vi "solar_voy_def Export (Mods).vi"(10 "CMD":enum8{"CMD", "TLM"}(ring), 11 "MODIFIERS":T1) -> (3 "MODIFIERS_DEF":string)   [LabVIEW 2018]
doc: "This exports a COSMOS parameter/item modifier to string."
uses:
  solar_voy_def_ctl MODIFIERS UNITS.ctl
  solar_voy_def_ctl MODIFIERS STATE.ctl
  solar_voy_def_ctl MODIFIERS CONVERSION.ctl
  solar_voy_def_ctl MODIFIERS.ctl
  solar_voy_def_ctl MODIFIERS LIMITS.ctl
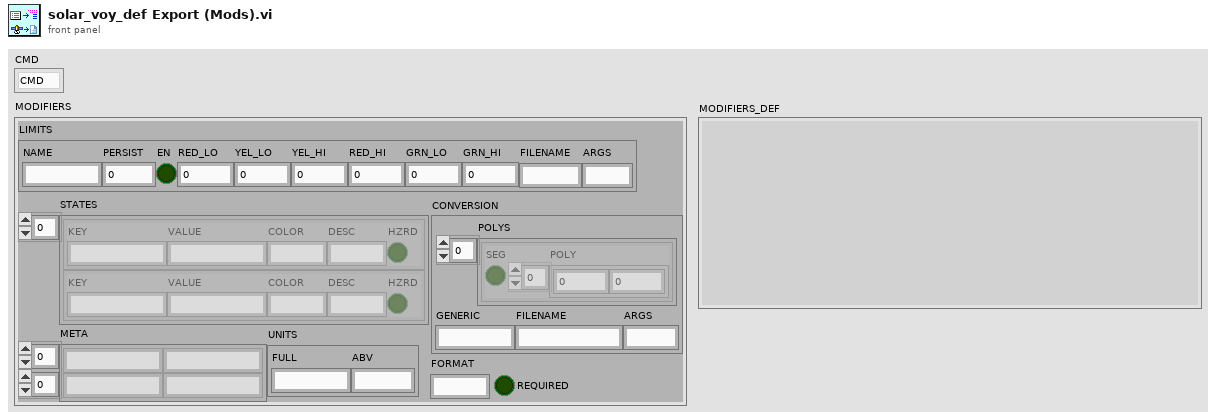
[diagram p1: front panel]
types:
  T1 = typedef "solar_voy_def_ctl MODIFIERS.ctl" = cluster{"LIMITS":T2, "UNITS":T3, "STATES":T4[], "CONVERSION":T5, "FORMAT":string, "REQUIRED":bool, "META":string[][]}
  T2 = typedef "solar_voy_def_ctl MODIFIERS LIMITS.ctl" = cluster{"NAME":string, "PERSIST":i32, "EN":bool, "RED_LO":dbl, "YEL_LO":dbl, "YEL_HI":dbl, "RED_HI":dbl, "GRN_LO":dbl, "GRN_HI":dbl, "FILENAME":string, "ARGS":string}
  T3 = typedef "solar_voy_def_ctl MODIFIERS UNITS.ctl" = cluster{"FULL":string, "ABV":string}
  T4 = typedef "solar_voy_def_ctl MODIFIERS STATE.ctl" = cluster{"KEY":string, "VALUE":string, "COLOR":string, "DESC":string, "HZRD":bool}
  T5 = typedef "solar_voy_def_ctl MODIFIERS CONVERSION.ctl" = cluster{"GENERIC":string, "FILENAME":string, "ARGS":string, "POLYS":cluster{"SEG":bool, "POLY":dbl[]}[]}
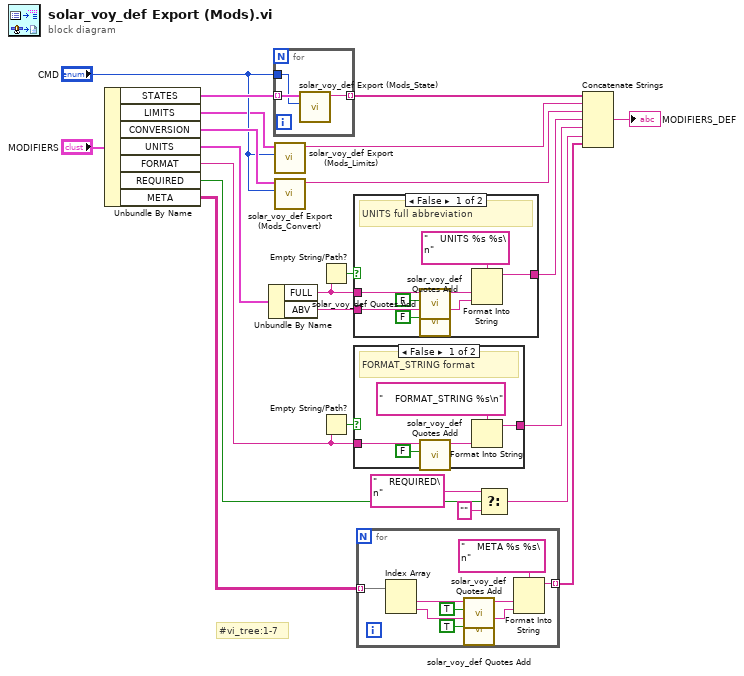
[diagram p0: block diagram]
diagram:
  # "#vi_tree:1-7"
  n1 = Unbundle By Name("MODIFIERS") -> ("STATES"=w22:T4[], "LIMITS"=w2:T2, "CONVERSION"=w19:T5, "UNITS"=w17:T3, "FORMAT"=w11:string, "REQUIRED"=w9:bool, "META"=w5:string[][])
  n2 = Unbundle By Name(w17) -> ("FULL"=w15:string, "ABV"=w14:string)
  n3 = for {
    tunnel: w22 -> [w25] mode=indexing
    tunnel: [w26] -> w21 mode=indexing
    tunnel: "CMD" -> [w24]
    n4 = call "solar_voy_def Export (Mods_State).vi"("CMD"=w24, "STATE"=w25) -> ("STATE_DEF"=w26:string)  [unwired: 9 in]
  }
  n5 = call "solar_voy_def Export (Mods_Limits).vi"("CMD"="CMD", "LIMITS"=w2) -> ("LIMITS_DEF"=w1:string)  [unwired: 9 in]
  n6 = call "solar_voy_def Export (Mods_Convert).vi"("CMD"="CMD", "CONVERSION"=w19) -> ("CONVERSION_DEF"=w18:string)  [unwired: 9 in]
  n7 = Empty String/Path?(string/path=w15) -> (empty?=w16:bool)
  n8 = Empty String/Path?(string/path=w11) -> (empty?=w12:bool)
  n9 = case shown="False" w16 {
    tunnel: w15 -> [w33 _]
    tunnel: w14 -> [w31 _]
    tunnel: [w27 _] -> w13
    frame False {
      # "UNITS full abbreviation"
      n10 = call "solar_voy_def Quotes Add.vi"("Whitespace Only? (F=Always)"=FALSE, "String"=w33) -> ("String with Comments"=w30:string)  [unwired: 9 in]
      n11 = call "solar_voy_def Quotes Add.vi"("Whitespace Only? (F=Always)"=FALSE, "String"=w31) -> ("String with Comments"=w29:string)  [unwired: 9 in]
      n12 = Format Into String(format string="    UNITS %s %s\n", w30, w29) -> (resulting string=w27:string)  [unwired: 2 in, 1 out]
    }
    frame True {
    }
  }
  n13 = case shown="False" w12 {
    tunnel: w11 -> [w38 _]
    tunnel: [w35 _] -> w10
    frame False {
      # "FORMAT_STRING format"
      n14 = call "solar_voy_def Quotes Add.vi"("Whitespace Only? (F=Always)"=FALSE, "String"=w38) -> ("String with Comments"=w37:string)  [unwired: 9 in]
      n15 = Format Into String(format string="    FORMAT_STRING %s\n", w37) -> (resulting string=w35:string)  [unwired: 2 in, 1 out]
    }
    frame True {
    }
  }
  n16 = for {
    tunnel: w5 -> [w48] mode=indexing
    tunnel: [w40] -> w4 mode=indexing
    n17 = Index Array(array=w48) -> (element #1=w45:string, element #2=w44:string)  [unwired: 2 in]
    n18 = call "solar_voy_def Quotes Add.vi"("Whitespace Only? (F=Always)"=TRUE, "String"=w45) -> ("String with Comments"=w43:string)  [unwired: 9 in]
    n19 = call "solar_voy_def Quotes Add.vi"("Whitespace Only? (F=Always)"=TRUE, "String"=w44) -> ("String with Comments"=w42:string)  [unwired: 9 in]
    n20 = Format Into String(format string="    META %s %s\n", w43, w42) -> (resulting string=w40:string)  [unwired: 2 in, 1 out]
  }
  n21 = Select(t="    REQUIRED\n", s=w9, f="") -> (s? t:f=w6:string)
  n22 = Concatenate Strings(w21, w1, w18, w13, w10, w6, w4) -> (→"MODIFIERS_DEF":string)
